vi "Configure Frequency.vi"(7 "Mode":enum16{"Center Span", "Start Stop"}(ring), 8 "error in (no error)":errorcluster, 9 "Span/Stop Frequency":dbl, 10 "Center/Start Frequency":dbl, 11 "VNA-ZNB in":refnum<class "VNA-ZNB.lvclass">) -> (0 "error out":errorcluster, 3 "VNA-ZNB out":refnum<class "VNA-ZNB.lvclass">)   [LabVIEW 2020, in "VNA-ZNB.lvclass"]
doc: "Configures the frequency range for the sweep.\nThe default mode is Center Span."
uses:
  VNA-ZNB.lvclass
  C:/Sandbox/Git_Sandbox/WiSpry Test Framework source code (LV20)/WiSpry Test Framework/Instruments/Vector Network Analyzer/Vector Network Analyzer.lvclass
  C:/Sandbox/Git_Sandbox/WiSpry Test Framework source code (LV20)/WiSpry Test Framework/Instruments/Instrument.lvclass
  Vector Network Analyzer.lvclass/Vector Network Analyzer.ctl
  Instrument.lvclass/Instrument.ctl
  Vector Network Analyzer.lvclass
  Instrument.lvclass
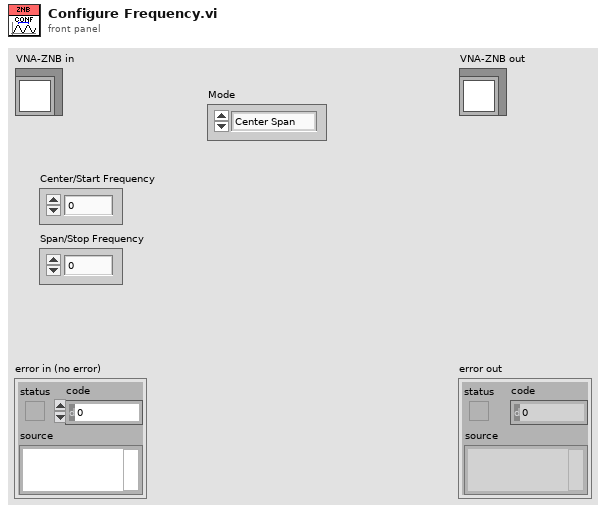
[diagram p1: front panel]
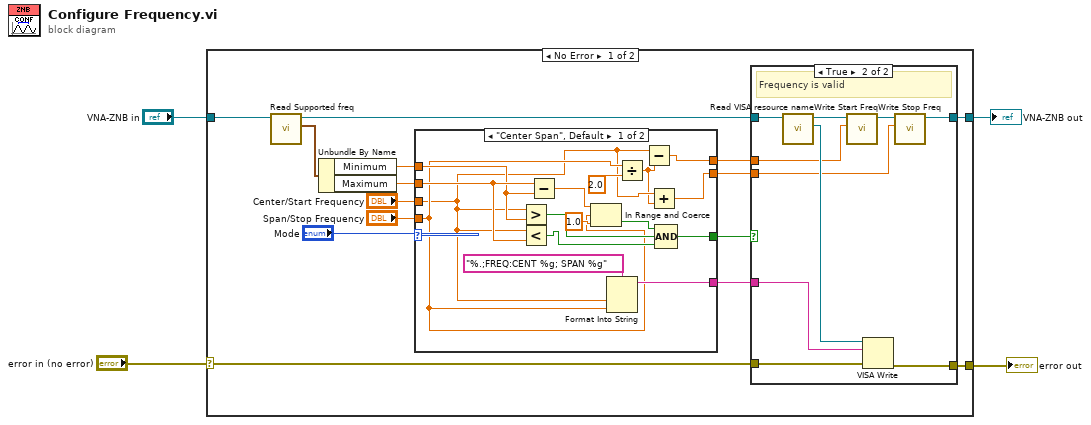
[diagram p0: block diagram]
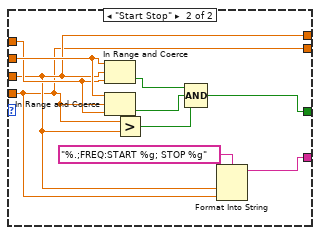
[diagram p3: hidden frame]
diagram:
  n1 = case shown="No Error" "error in (no error)" {
    selector: "error in (no error)" -> [w9 w58]
    tunnel: "VNA-ZNB in" -> [w19 w59]
    tunnel: [w8 w59] -> w2
    tunnel: [w7 w58] -> w1
    frame No Error {
      n2 = call "Read Supported freq.vi"("Vector Network Analyzer in"=w19) -> ("Supported freq"=w18:cluster{"Minimum":dbl, "Maximum":dbl}, "Vector Network Analyzer out"=w10:refnum<class "VNA-ZNB.lvclass">)  [unwired: 9 in]
      n3 = Unbundle By Name(w18) -> ("Minimum"=w17:dbl, "Maximum"=w16:dbl)
      n4 = case shown="\"Center Span\", Default" "Mode" {
        tunnel: w17 -> [w46 w50]
        tunnel: w16 -> [w47 w57]
        tunnel: "Center/Start Frequency" -> [w34 w49]
        tunnel: "Span/Stop Frequency" -> [w36 w48]
        tunnel: [w41 w53] -> w12
        tunnel: [w39 w51] -> w11
        tunnel: [w35 w49] -> w6
        tunnel: [w32 w48] -> w5
        frame "Center Span", Default {
          n5 = Greater?(x=w34, y=w46) -> (0:w43:bool)
          n6 = Less?(x=w34, y=w47) -> (x < y?=w42:bool)
          n7 = Subtract(x=w47, y=w46) -> (x-y=w38:dbl)
          n8 = In Range and Coerce(upper limit=w38, x=w36, lower limit=1.0) -> (In Range?=w44:bool)  [unwired: 1 out]
          n9 = Format Into String(format string="%.;FREQ:CENT %g; SPAN %g", w34, w36) -> (resulting string=w39:string)  [unwired: 2 in, 1 out]
          n10 = Divide(x=w36, y=2.0) -> (x/y=w33:dbl)
          n11 = Subtract(x=w34, y=w33) -> (x-y=w35:dbl)
          n12 = Add(x=w34, y=w33) -> (x+y=w32:dbl)
          n13 = Compound Arithmetic op=AND(w44, w43, w42) -> (w41:bool)
        }
        frame "Start Stop" {
          n14 = In Range and Coerce(upper limit=w57, x=w49, lower limit=w50) -> (In Range?=w56:bool)  [unwired: 1 out]
          n15 = In Range and Coerce(upper limit=w57, x=w48, lower limit=w50) -> (In Range?=w55:bool)  [unwired: 1 out]
          n16 = Greater?(x=w48, y=w49) -> (0:w54:bool)
          n17 = Compound Arithmetic op=AND(w56, w55, w54) -> (w53:bool)
          n18 = Format Into String(format string="%.;FREQ:START %g; STOP %g", w49, w48) -> (resulting string=w51:string)  [unwired: 2 in, 1 out]
        }
      }
      n19 = case shown="True" w12 {
        tunnel: w11 -> [_ w30]
        tunnel: w10 -> [w21 w29]
        tunnel: w9 -> [w20 w31]
        tunnel: [w21 w23] -> w8
        tunnel: [w20 w27] -> w7
        tunnel: w6 -> [_ w25]
        tunnel: w5 -> [_ w22]
        frame False {
          # "Add error handler"
          # "Frequency not valid"
        }
        frame True {
          # "Frequency is valid"
          n20 = call "Read VISA resource name.vi"("Instrument in"=w29) -> ("VISA resource name"=w28:refnum<visa-resource-name>, "Instrument out"=w26:refnum<class "VNA-ZNB.lvclass">)  [unwired: 9 in]
          n21 = call "Write Start Freq.vi"("Start Freq"=w25, "Vector Network Analyzer in"=w26) -> ("Vector Network Analyzer out"=w24:refnum<class "VNA-ZNB.lvclass">)  [unwired: 9 in]
          n22 = VISA Write(VISA resource name=w28, write buffer=w30, error in (no error)=w31) -> (error out=w27:errorcluster)  [unwired: 2 out]
          n23 = call "Write Stop Freq.vi"("Stop Freq"=w22, "Vector Network Analyzer in"=w24) -> ("Vector Network Analyzer out"=w23:refnum<class "VNA-ZNB.lvclass">)  [unwired: 9 in]
        }
      }
    }
    frame Error {
    }
  }
  "error out" <- w1
  "VNA-ZNB out" <- w2
